vi "AcqWait.vi"(2 "error in":errorcluster, 3 "ActXDSO In":refnum<k7>) -> (0 "error out":errorcluster, 1 "ActXDSO Out":refnum<k7>)   [LabVIEW 2022 SP3]
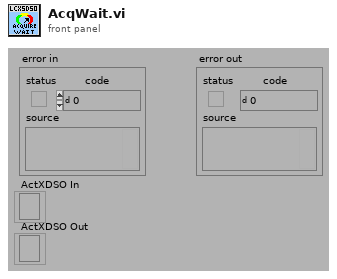
[diagram p1: front panel]
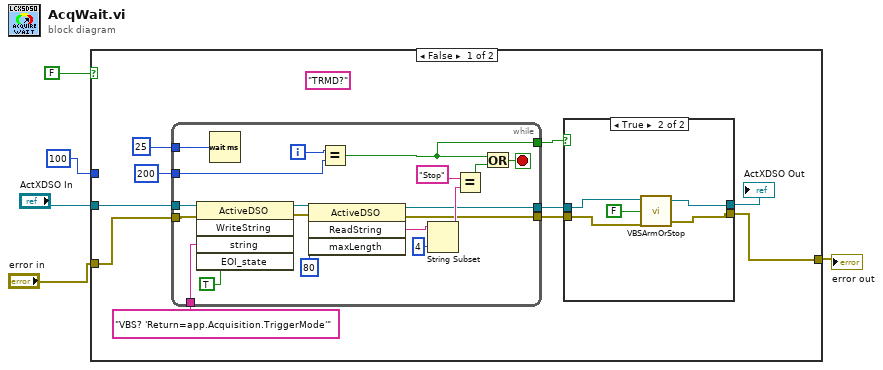
[diagram p0: block diagram]
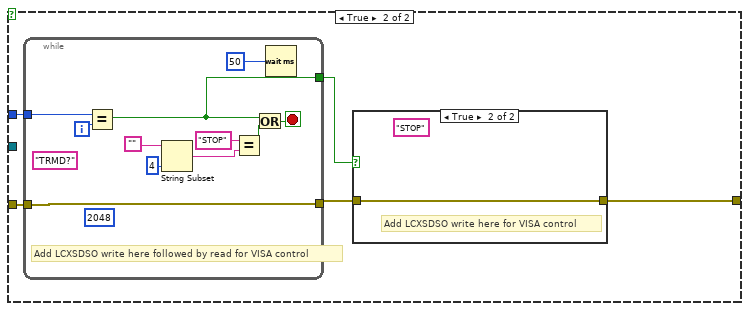
[diagram p3: hidden frame]
diagram:
  n1 = case shown="False" FALSE ("Case Constant\n(See Context Help)") {
    tunnel: "error in" -> [w12 w46]
    tunnel: [w7 w44] -> w4
    tunnel: 100 -> [_ w42]
    tunnel: "ActXDSO In" -> [w8 _]
    frame False {
      (unwired) "TRMD?"
      n2 = while {
        tunnel: "VBS? 'Return=app.Acquisition.TriggerMode'" -> [w34]
        tunnel: 25 -> [w33]
        tunnel: 200 -> [w31]
        tunnel: w8 -> [w30]
        tunnel: w12 -> [w29]
        tunnel: [w23] -> w11
        tunnel: [w22] -> w10
        tunnel: [w19] -> w9
        i -> [w32]
        stop <- w20 stop-if-true
        n3 = invoke class="ActiveDSO" method="WriteString"(reference=w30, error in=w29, "string"=w34, "EOI_state"=TRUE) -> (reference out=w28:refnum<k7>, error out=w27:errorcluster)  [unwired: 1 in, 3 out]
        n4 = Wait (ms)(milliseconds to wait=w33) -> ()  [unwired: 1 out]
        n5 = invoke class="ActiveDSO" method="ReadString"(reference=w28, error in=w27, "maxLength"=80) -> (reference out=w23:refnum<k7>, error out=w22:errorcluster, "ReadString"=w24:string)  [unwired: 1 in, 1 out]
        n6 = Equal?(x=w32, y=w31) -> (x = y?=w19:bool)
        n7 = String Subset(string=w24, length (rest)=4) -> (substring=w25:string)  [unwired: 1 out]
        n8 = Equal?(x="Stop", y=w25) -> (x = y?=w21:bool)
        n9 = Or(x=w19, y=w21) -> (x .or. y?=w20:bool)
      }
      n10 = case shown="True" w9 {
        tunnel: [w36 w38] -> w7
        tunnel: w11 -> [w35 w40]
        tunnel: w10 -> [w36 w39]
        tunnel: [w35 w37] -> w6
        frame False {
        }
        frame True {
          n11 = call "VBSArmOrStop.vi"("error in (no error)"=w39, "Arm T/Stop F"=FALSE, "ActXDSO In"=w40) -> ("error out"=w38:errorcluster, "ActXDSO Out"=w37:refnum<k7>)  [unwired: 1 out]
        }
      }
      "ActXDSO Out" <- w6
    }
    frame True {
      n12 = while {
        tunnel: w46 -> [w50]
        tunnel: [w50] -> w43
        tunnel: [w52] -> w45
        tunnel: w42 -> [w51]
        i -> [w58]
        stop <- w57 stop-if-true
        (unwired) "TRMD?"
        (unwired) 2048
        # "Add LCXSDSO write here followed by read for VISA control"
        n13 = Equal?(x=w51, y=w58) -> (x = y?=w52:bool)
        n14 = String Subset(string="", length (rest)=4) -> (substring=w54:string)  [unwired: 1 out]
        n15 = Equal?(x="STOP", y=w54) -> (x = y?=w55:bool)
        n16 = Or(x=w52, y=w55) -> (x .or. y?=w57:bool)
        n17 = Wait (ms)(milliseconds to wait=50) -> ()  [unwired: 1 out]
      }
      n18 = case shown="True" w45 {
        tunnel: [w47 w48] -> w44
        tunnel: w43 -> [w47 w48]
        frame False {
        }
        frame True {
          (unwired) "STOP" ("write buffer")
          # "Add LCXSDSO write here for VISA control"
        }
      }
    }
  }
  "error out" <- w4
